vi "Examen1.vi"() -> ()   [LabVIEW 2020]
uses:
  <vilib>/Analysis/Matrix/Datatypes/RealMatrix.ctl
  <vilib>/Analysis/Matrix/NI_Matrix.lvlib
panel:
  out "Comprobacion 2":string
  out "Array 3":dbl[](array[numeric])
  out "con1":dbl
  out "Comprobacion":string
  out "condicion":i32
  out "SG":dbl
  out "element":dbl
  out "Diago1":dbl[](array[numeric])
  out "Suma Columnas":dbl[](array[numeric])
  out "Suma Filas":dbl[](array[numeric])
  out "DIAGO2":dbl
  out "tamañoo":i32
  in  "Real Matrix":T1
  out "TOTAL":dbl
  out "Numeric":i16
  out "SG":dbl
  out "1Diagonal":i32
  out "2Diagonal":i16
  out "Array 2":dbl[](array[numeric])
  in  "index":i16
  out "SUMA COLUMNAS":dbl[](array[numeric])
  out "AUXI 2":dbl[](array[numeric])
  out "SUMA FILAS":dbl[](array[numeric])
  out "AUXI":dbl[](array[numeric])
  out "Array":u16[][](array[numeric])
  in  "n":i16
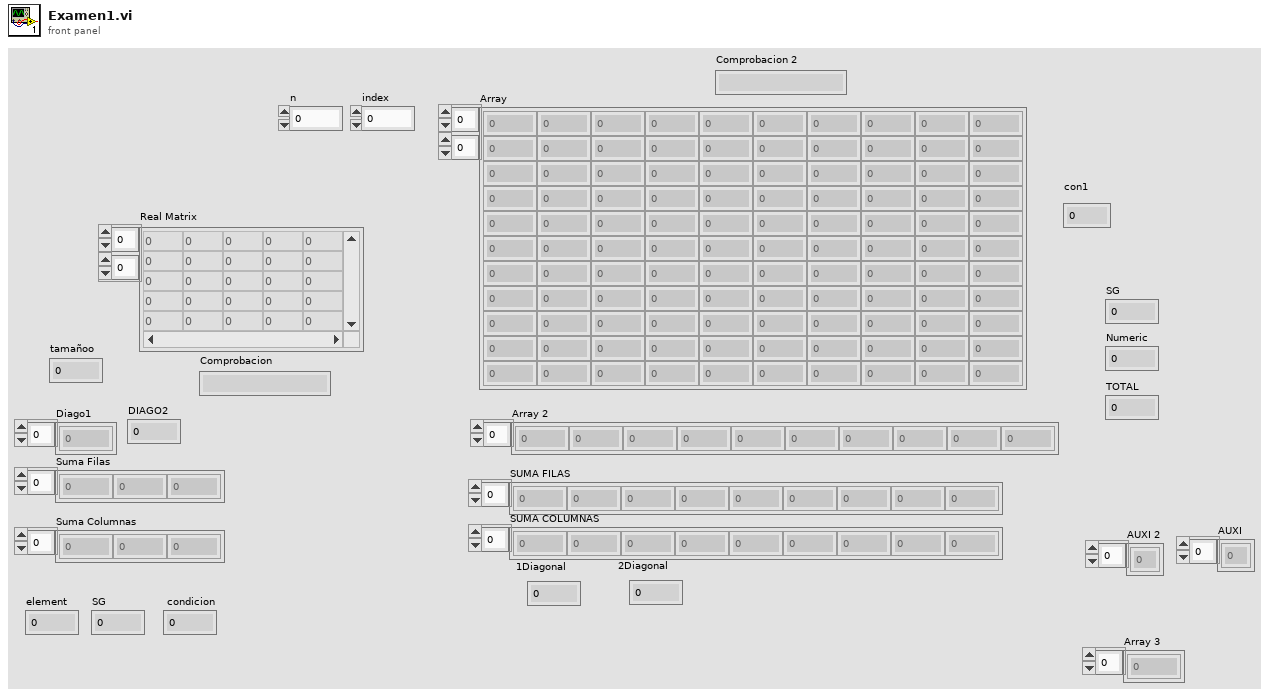
[diagram p1: front panel]
types:
  T1 = typedef "NI_Matrix.lvlib/RealMatrix.ctl" = dbl[][]
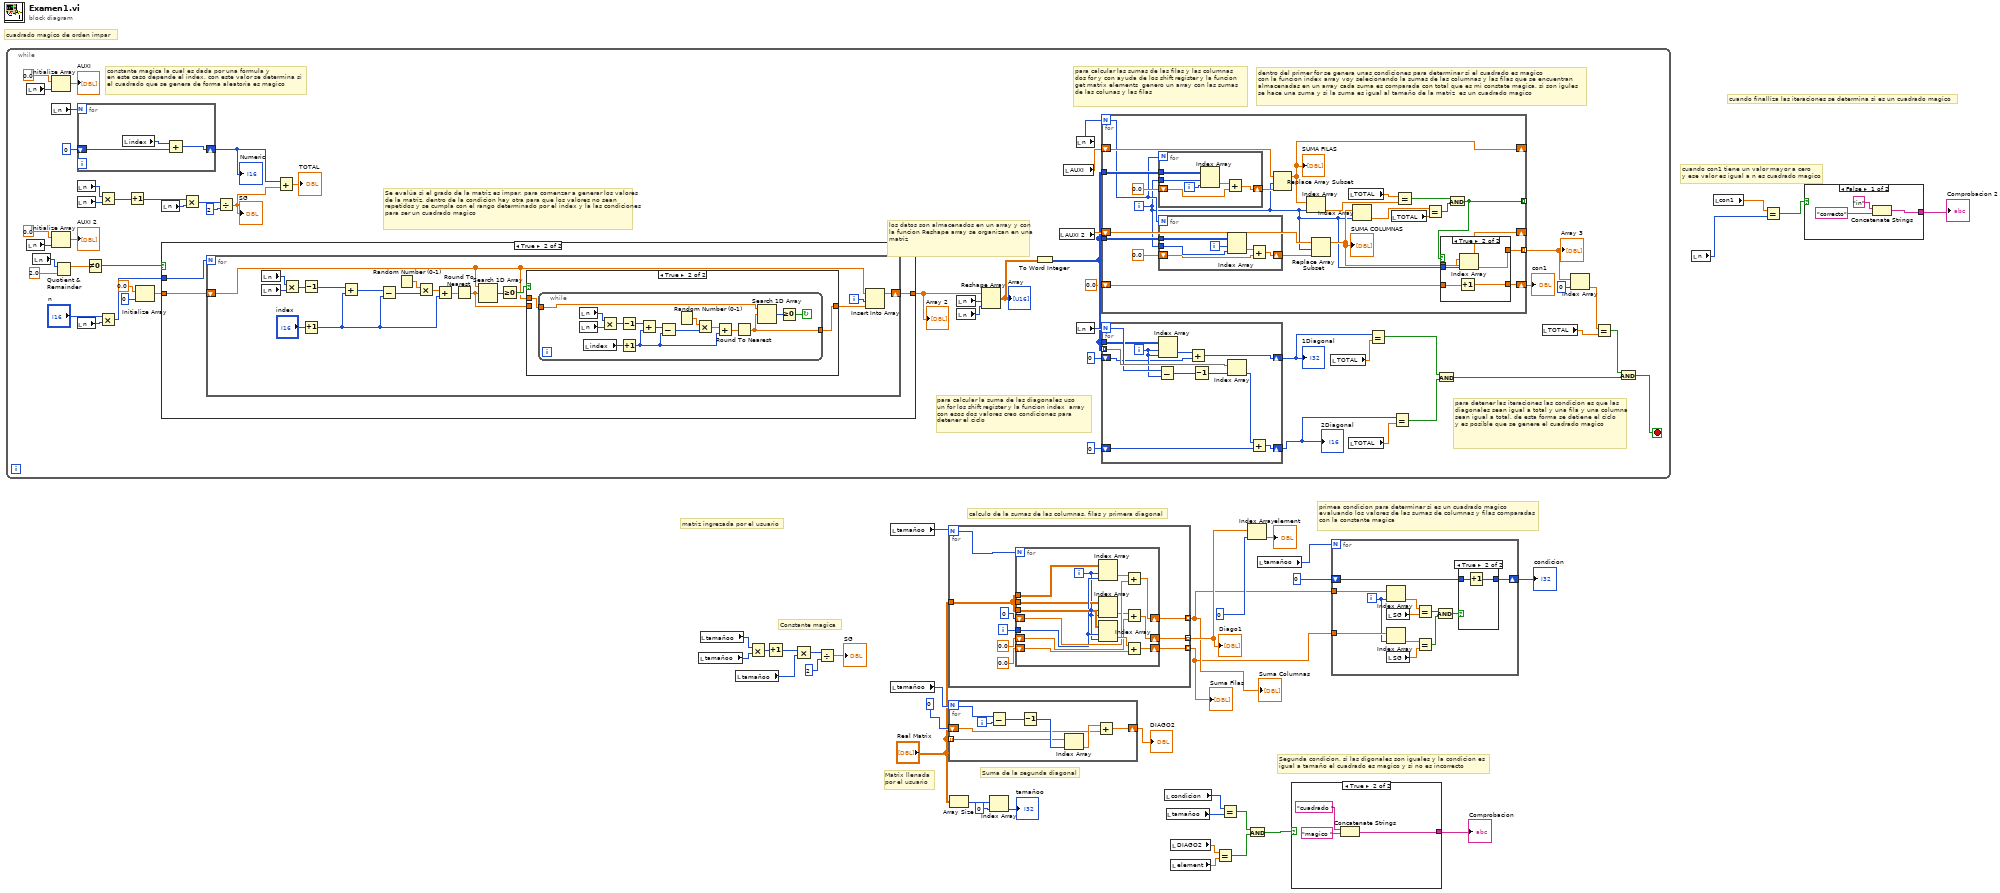
[diagram p0: block diagram]
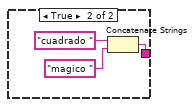
[diagram p2: hidden frame]
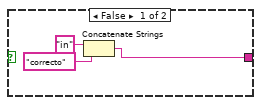
[diagram p3: hidden frame]
diagram:
  # "cuando con1 tiene un valor mayor a cero\ny ese valor es igual a n es cuadrado magico"
  # "matriz ingrezada por el usuario"
  # "cuadrado magico de orden impar"
  # "cuando finalliza las iteraciones se determina si es un cuadrado magico"
  # "Segunda condicion, si las digonales son iguales y la condicion es \nigual a tamaño el cuadrado es magico y si no es incorrecto"
  # "primea condicion para determinar si es un cuadrado magico \nevaluando los valores de las sumas de columnas y filas comparadas \ncon la constante magica"
  # "Suma de la segunda diagonal"
  # "calculo de la sumas de las columnas, filas y primera diagonal"
  # "Matrix llenada \npor el usuario"
  # "Constante magica"
  n1 = while {
    stop <- w38 stop-if-true
    # "para detener las iteraciones las condicion es que las \ndiagonales sean igual a total y una fila y una columna \nsean igual a total, de esta forma se detiene el ciclo \ny es posible que se genere el cuadrado magico"
    # "para calcular la suma de las diagonales uso \nun for los shift register y la funcion index  array \ncon esos dos valores creo condiciones para \ndetener el ciclo"
    # "dentro del primer for se genera unas condiciones para determinar si el cuadrado es magico \ncon la funcion index array voy selecionando la sumas de las columnas y las filas que se encuentran \nalmacenadas en un array cada suma es comparada con total que es mi constate magica, si son igules \nse hace una suma y si la suma es igual al tamaño de la matriz  es un cuadrado magico"
    # "para calcular las sumas de las filas y las columnas \ndos for y con ayuda de los shift register y la funcion\nget matrix elements  genero un array con las sumas \nde las colunas y las filas"
    # "los datos son almacenados en un array y con la funcion Reshape array se organizan en una matriz"
    # "Se evalúa si el grado de la matriz es impar, para comenzar a generar los valores de la matriz, dentro de la condicion hay otra para que los valores no sean repetidos y se cumpla con el rango determinado por el index y la las condiciones para ser un cuadrado magico"
    # "constante magica la cual es dada por una formula y \nen este caso depende el index, con este valor se determina si \nel cuadrado que se genera de forma aleatoria es magico"
    n2 = local read "n"() -> (w89:i16)
    n3 = local read "n"() -> (w83:i16)
    n4 = local read "n"() -> (w79:i16)
    n5 = Initialize Array(0.0 ("element"), w89) -> (→"AUXI":dbl[])
    n6 = Initialize Array(0.0 ("element"), w83) -> (→"AUXI 2":dbl[])
    n7 = local read "n"() -> (w56:i16)
    n8 = Quotient & Remainder(x=w79, y=2.0) -> (x-y*floor(x/y)=w81:dbl)  [unwired: 1 out]
    n9 = for {
      N: w56 -> [_]
      shift-right: [w93] -> w54
      shift-left: i16 0 -> [w91]
      n10 = local read "index"() -> (w92:i16)
      n11 = Add(x=w92, y=w91) -> (x+y=w93:i16)
    }
    "Numeric" <- w54
    n12 = local read "n"() -> (w63:i16)
    n13 = local read "n"() -> (w62:i16)
    n14 = local read "n"() -> (w74:i16)
    n15 = Not Equal To 0?(x=w81) -> (x != 0?=w76:bool)
    n16 = Multiply(x=w63, y=w62) -> (x*y=w61:i16)
    n17 = Multiply(x="n", y=w74) -> (x*y=w73:i16)
    n18 = Increment(x=w61) -> (x+1=w60:i16)
    n19 = Initialize Array(0.0 ("element"), 0 ("dimension size")) -> (w72:dbl[])
    n20 = local read "n"() -> (w59:i16)
    n21 = case shown="True" w76 {
      tunnel: w73 -> [_ w96]
      tunnel: w72 -> [_ w95]
      tunnel: [_ w94] -> w69
      frame False {
      }
      frame True {
        n22 = for {
          N: w96 -> [_]
          shift-right: [w100] -> w94
          shift-left: w95 -> [w99]
          i -> [w97]
          n23 = local read "n"() -> (w106:i16)
          n24 = local read "n"() -> (w105:i16)
          n25 = Multiply(x=w106, y=w105) -> (x*y=w108:i16)
          n26 = Decrement(x=w108) -> (x-1=w107:i16)
          n27 = Increment(x="index") -> (x+1=w110:i16)
          n28 = Add(x=w107, y=w110) -> (x+y=w109:i16)
          n29 = Subtract(x=w109, y=w110) -> (x-y=w112:i16)
          n30 = Random Number (0-1)() -> (number: 0 to 1=w113:dbl)
          n31 = Multiply(x=w113, y=w112) -> (x*y=w111:dbl)
          n32 = Add(x=w111, y=w110) -> (x+y=w104:dbl)
          n33 = Round To Nearest(number=w104) -> (nearest integer value=w98:dbl)
          n34 = Search 1D Array(1D array=w99, element=w98) -> (index of element=w103:i32)  [unwired: 1 in]
          n35 = Greater Or Equal To 0?(x=w103) -> (x >= 0?=w102:bool)
          n36 = case shown="True" w102 {
            tunnel: [w115 w117] -> w101
            tunnel: w99 -> [_ w116]
            tunnel: w98 -> [w115 _]
            frame False {
            }
            frame True {
              n37 = while {
                tunnel: [w121] -> w117
                tunnel: w116 -> [w120]
                stop <- w119 continue-if-true
                n38 = local read "n"() -> (w123:i16)
                n39 = local read "n"() -> (w122:i16)
                n40 = local read "index"() -> (w118:i16)
                n41 = Multiply(x=w123, y=w122) -> (x*y=w127:i16)
                n42 = Decrement(x=w127) -> (x-1=w126:i16)
                n43 = Increment(x=w118) -> (x+1=w129:i16)
                n44 = Add(x=w126, y=w129) -> (x+y=w128:i16)
                n45 = Subtract(x=w128, y=w129) -> (x-y=w131:i16)
                n46 = Random Number (0-1)() -> (number: 0 to 1=w132:dbl)
                n47 = Multiply(x=w132, y=w131) -> (x*y=w130:dbl)
                n48 = Add(x=w130, y=w129) -> (x+y=w125:dbl)
                n49 = Round To Nearest(number=w125) -> (nearest integer value=w121:dbl)
                n50 = Search 1D Array(1D array=w120, element=w121) -> (index of element=w124:i32)  [unwired: 1 in]
                n51 = Greater Or Equal To 0?(x=w124) -> (x >= 0?=w119:bool)
              }
            }
          }
          n52 = Insert Into Array(array=w99, index=w97, new element=w101) -> (w100:dbl[])
        }
      }
    }
    "Array 2" <- w69
    n53 = Multiply(x=w60, y=w59) -> (x*y=w58:i16)
    n54 = Divide(x=w58, y=i16 2) -> (x/y=w53:dbl)
    "SG" <- w53
    n55 = Add(x=w54, y=w53) -> (x+y=→"TOTAL":dbl)
    n56 = local read "n"() -> (w68:i16)
    n57 = local read "n"() -> (w67:i16)
    n58 = Reshape Array(w69, w68, w67) -> (w66:dbl[][])
    "Array" <- w66
    n59 = To Word Integer(number=w66) -> (16bit integer=w77:i16[][])
    n60 = local read "AUXI 2"() -> (w82:dbl[])
    n61 = local read "AUXI"() -> (w86:dbl[])
    n62 = local read "n"() -> (w90:i16)
    n63 = local read "n"() -> (w78:i16)
    n64 = for {
      N: w90 -> [w162]
      tunnel: w77 -> [w166]
      shift-right: [w157] -> _
      shift-left: w86 -> [w164]
      tunnel: w77 -> [w161]
      shift-right: [w147] -> _
      shift-left: w82 -> [w159]
      shift-right: [w149] -> w49
      shift-left: 0.0 -> [w150]
      tunnel: [w148] -> _ mode=indexing
      tunnel: [w145] -> w43 mode=indexing
      i -> [w146]
      n65 = for {
        N: w162 -> [_]
        tunnel: w166 -> [w183]
        tunnel: w146 -> [w182]
        shift-right: [w179] -> w163
        shift-left: 0.0 -> [w178]
        i -> [w181]
        n66 = Index Array(array=w183, index (row)=w182, index (col)=w181) -> (element=w180:dbl)
        n67 = Add(x=w180, y=w178) -> (x+y=w179:dbl)
      }
      n68 = for {
        N: w162 -> [_]
        tunnel: w161 -> [w177]
        tunnel: w146 -> [w175]
        shift-right: [w173] -> w158
        shift-left: 0.0 -> [w172]
        i -> [w176]
        n69 = Index Array(array=w177, index (row)=w176, index (col)=w175) -> (element=w174:dbl)
        n70 = Add(x=w174, y=w172) -> (x+y=w173:dbl)
      }
      n71 = Replace Array Subset(array=w164, new element=w163, index=w146) -> (w157:dbl[])
      "SUMA FILAS" <- w157
      n72 = Index Array(array=w157, index=w146) -> (element=w155:dbl)
      n73 = Replace Array Subset(array=w159, new element=w158, index=w146) -> (w147:dbl[])
      "SUMA COLUMNAS" <- w147
      n74 = local read "TOTAL"() -> (w156:dbl)
      n75 = Index Array(array=w147, index=w146) -> (element=w154:dbl)
      n76 = local read "TOTAL"() -> (w153:dbl)
      n77 = Equal?(x=w156, y=w155) -> (x = y?=w152:bool)
      n78 = Equal?(x=w154, y=w153) -> (x = y?=w151:bool)
      n79 = And(x=w152, y=w151) -> (x .and. y?=w148:bool)
      n80 = case shown="True" w148 {
        tunnel: w150 -> [_ w171]
        tunnel: [_ w170] -> w149
        tunnel: w147 -> [_ w169]
        tunnel: w146 -> [_ w168]
        tunnel: [_ w167] -> w145
        frame False {
        }
        frame True {
          n81 = Increment(x=w171) -> (x+1=w170:dbl)
          n82 = Index Array(array=w169, index=w168) -> (element=w167:dbl)
        }
      }
    }
    "con1" <- w49
    "Array 3" <- w43
    n83 = for {
      N: w78 -> [w141]
      tunnel: w77 -> [w137]
      tunnel: w77 -> [w144] mode=indexing
      shift-right: [w139] -> w47
      shift-left: i16 0 -> [w138]
      shift-right: [w133] -> w51
      shift-left: 0 -> [w134]
      i -> [w136]
      n84 = Subtract(x=w141, y=w136) -> (x-y=w143:i32)
      n85 = Index Array(array=w137, index (row)=w136, index (col)=w136) -> (element=w135:i16)
      n86 = Add(x=w135, y=w134) -> (x+y=w133:i32)
      n87 = Decrement(x=w143) -> (x-1=w142:i32)
      n88 = Index Array(array=w144, index=w142) -> (element=w140:i16)
      n89 = Add(x=w140, y=w138) -> (x+y=w139:i16)
    }
    "2Diagonal" <- w47
    "1Diagonal" <- w51
    n90 = local read "TOTAL"() -> (w48:dbl)
    n91 = local read "TOTAL"() -> (w46:dbl)
    n92 = Equal?(x=w51, y=w48) -> (x = y?=w45:bool)
    n93 = Equal?(x=w47, y=w46) -> (x = y?=w44:bool)
    n94 = And(x=w45, y=w44) -> (x .and. y?=w39:bool)
    n95 = local read "TOTAL"() -> (w40:dbl)
    n96 = Index Array(array=w43, index=0) -> (element=w41:dbl)
    n97 = Equal?(x=w41, y=w40) -> (x = y?=w37:bool)
    n98 = And(x=w37, y=w39) -> (x .and. y?=w38:bool)
  }
  n99 = local read "tamañoo"() -> (w21:i32)
  n100 = local read "tamañoo"() -> (w22:i32)
  n101 = local read "tamañoo"() -> (w19:i32)
  n102 = Multiply(x=w22, y=w21) -> (x*y=w20:i32)
  n103 = Increment(x=w20) -> (x+1=w18:i32)
  n104 = Multiply(x=w18, y=w19) -> (x*y=w17:i32)
  n105 = Divide(x=w17, y=2) -> (x/y=→"SG":dbl)
  n106 = local read "tamañoo"() -> (w29:i32)
  n107 = local read "tamañoo"() -> (w33:i32)
  n108 = for {
    N: w29 -> [w189]
    tunnel: "Real Matrix" -> [w186]
    tunnel: [w190] -> w23 mode=indexing
    tunnel: [w187] -> w24 mode=indexing
    tunnel: [w184] -> w28 mode=indexing
    i -> [w192]
    n109 = for {
      N: w189 -> [_]
      tunnel: w186 -> [w206]
      tunnel: w192 -> [w198]
      shift-right: [w203] -> w190
      shift-left: 0.0 -> [w204]
      tunnel: w186 -> [w202]
      shift-right: [w199] -> w187
      shift-left: 0 -> [w200]
      tunnel: w186 -> [w197]
      shift-right: [w194] -> w184
      shift-left: 0.0 -> [w195]
      i -> [w193]
      n110 = Index Array(array=w202, index (row)=w193, index (col)=w198) -> (element=w201:dbl)
      n111 = Index Array(array=w197, index (row)=w193, index (col)=w193) -> (element=w196:dbl)
      n112 = Index Array(array=w206, index (row)=w198, index (col)=w193) -> (element=w205:dbl)
      n113 = Add ("Add.vi")(x=w201, y=w200) -> (x+y=w199:dbl)
      n114 = Add ("Add.vi")(x=w196, y=w195) -> (x+y=w194:dbl)
      n115 = Add ("Add.vi")(x=w205, y=w204) -> (x+y=w203:dbl)
    }
  }
  "Suma Filas" <- w23
  "Suma Columnas" <- w24
  "Diago1" <- w28
  n116 = for {
    N: w33 -> [w212]
    tunnel: "Real Matrix" -> [w208] mode=indexing
    shift-right: [w209] -> w31
    shift-left: 0 -> [w210]
    i -> [w207]
    n117 = Subtract(x=w212, y=w207) -> (x-y=w214:i32)
    n118 = Decrement(x=w214) -> (x-1=w213:i32)
    n119 = Index Array(array=w208, index=w213) -> (element=w211:dbl)
    n120 = Add(x=w211, y=w210) -> (x+y=w209:dbl)
  }
  "DIAGO2" <- w31
  n121 = Array Size(array="Real Matrix") -> (size(s)=w36:i32[])
  n122 = Index Array(array=w36, index=0) -> (element=→"tamañoo":i32)
  n123 = local read "condicion"() -> (w12:i32)
  n124 = local read "tamañoo"() -> (w11:i32)
  n125 = local read "DIAGO2"() -> (w9:dbl)
  n126 = local read "element"() -> (w8:dbl)
  n127 = Equal?(x=w9, y=w8) -> (x = y?=w6:bool)
  n128 = Equal?(x=w12, y=w11) -> (x = y?=w7:bool)
  n129 = Index Array(array=w28, index=0) -> (element=→"element":dbl)
  n130 = And(x=w7, y=w6) -> (x .and. y?=w5:bool)
  n131 = local read "tamañoo"() -> (w25:i32)
  n132 = case shown="True" w5 {
    tunnel: [w215 w218] -> w10
    frame False {
      n133 = Concatenate Strings("in" ("string"), "correcto" ("string")) -> (w215:string)
    }
    frame True {
      n134 = Concatenate Strings("cuadrado " ("string"), "magico " ("string")) -> (w218:string)
    }
  }
  "Comprobacion" <- w10
  n135 = for {
    N: w25 -> [_]
    tunnel: w24 -> [w232]
    tunnel: w23 -> [w231]
    shift-right: [w221] -> w13
    shift-left: 0 -> [w222]
    i -> [w230]
    n136 = Index Array(array=w232, index=w230) -> (element=w229:dbl)
    n137 = Index Array(array=w231, index=w230) -> (element=w227:dbl)
    n138 = local read "SG"() -> (w228:dbl)
    n139 = local read "SG"() -> (w226:dbl)
    n140 = Equal?(x=w229, y=w228) -> (x = y?=w225:bool)
    n141 = Equal?(x=w227, y=w226) -> (x = y?=w224:bool)
    n142 = And(x=w225, y=w224) -> (x .and. y?=w223:bool)
    n143 = case shown="True" w223 {
      tunnel: w222 -> [_ w234]
      tunnel: [_ w233] -> w221
      frame False {
      }
      frame True {
        n144 = Increment(x=w234) -> (x+1=w233:i32)
      }
    }
  }
  "condicion" <- w13
  n145 = local read "n"() -> (w2:i16)
  n146 = local read "con1"() -> (w1:dbl)
  n147 = Equal?(x=w1, y=w2) -> (x = y?=w4:bool)
  n148 = case shown="False" w4 {
    tunnel: [w235 w238] -> w3
    frame False {
      n149 = Concatenate Strings("in" ("string"), "correcto" ("string")) -> (w235:string)
    }
    frame True {
      n150 = Concatenate Strings("cuadrado " ("string"), "magico " ("string")) -> (w238:string)
    }
  }
  "Comprobacion 2" <- w3
